vi "niDTS BT UTIL Parameters to Recepie.vi"(10 "BT Tx Parameters":T1={"Channel"=0, "Data Rate "=1, "Dut Tx Power"=0.0, "External Attenuation (dB)"=[0.0, 0.0, 0.0, 0.0], "Auto Level"=FALSE, "Packet type"=enum."DH1", "Payload Pattern"=enum."PN9", "Burst Sync"=enum."PREamble", "BD ADDRESS"=0, "Packet Length, bytes"=37, "ModAcc Measurement Paramaters"={"ModAcc Enable"=FALSE, "CFO Enable"=FALSE, "Character Select"=enum."DF1", "Averages"=1, "Averaging Mode"=enum."RMS", "Measurement Length"=-1, "Measurement Offset"=0}, "OBW Measurement Parameters"={"OBW Enable"=FALSE, "OBW Averages"=1, "Averaging Type"=enum."RMS", "Measurement Interval Mode"=enum."AUTO", "Measurement Interval Length (sec)"=0.005}, "TXP Measurement Parameters"={"TXP Power Enable"=FALSE, "TXP Averages"=1, "Averaging Type"=enum."RMS"}, "IBE  Measurement Parameters"={"IBE Enable"=FALSE, "IBE Averages"=1, "Averaging Type"=enum."RMS", "Numbe of Channels"=11, "Channel Mode"=enum."Centered", "Measurement Interval Mode"=enum."AUTO", "Measurement Interval Length (sec)"=0.005}, "Trace Enable"=FALSE, "Trigger"={"MinQuietTimeDuration (sec)"=0.0001, "TriggerDelay (sec)"=0.0, "TriggerEdge"=enum."RISing", "TriggerSource"=enum."RF0", "TriggerThreshold (dB)"=-20.0, "TriggerTimeout (sec)"=10.0}} {"BD ADDRESS" max=16777215 format="%.0x"}) -> (2 "BT Tx Parameters Out":T1={"Channel"=0, "Data Rate "=1, "Dut Tx Power"=0.0, "External Attenuation (dB)"=[0.0, 0.0, 0.0, 0.0], "Auto Level"=FALSE, "Packet type"=enum."DH1", "Payload Pattern"=enum."PN9", "Burst Sync"=enum."PREamble", "BD ADDRESS"=0, "Packet Length, bytes"=-1, "ModAcc Measurement Paramaters"={"ModAcc Enable"=FALSE, "CFO Enable"=FALSE, "Character Select"=enum."DF1", "Averages"=1, "Averaging Mode"=enum."RMS", "Measurement Length"=-1, "Measurement Offset"=0}, "OBW Measurement Parameters"={"OBW Enable"=FALSE, "OBW Averages"=1, "Averaging Type"=enum."RMS", "Measurement Interval Mode"=enum."AUTO", "Measurement Interval Length (sec)"=0.005}, "TXP Measurement Parameters"={"TXP Power Enable"=FALSE, "TXP Averages"=1, "Averaging Type"=enum."RMS"}, "IBE  Measurement Parameters"={"IBE Enable"=FALSE, "IBE Averages"=1, "Averaging Type"=enum."RMS", "Numbe of Channels"=11, "Channel Mode"=enum."Centered", "Measurement Interval Mode"=enum."AUTO", "Measurement Interval Length (sec)"=0.005}, "Trace Enable"=FALSE, "Trigger"={"MinQuietTimeDuration (sec)"=0.0001, "TriggerDelay (sec)"=0.0, "TriggerEdge"=enum."RISing", "TriggerSource"=enum."RF0", "TriggerThreshold (dB)"=-20.0, "TriggerTimeout (sec)"=10.0}} {"BD ADDRESS" max=16777215 format="%.0x"}, 4 "Payloads":T3[](array[typedef]), 5 "Measurements":enum16{"Other", "DF1", "DF2"}[](array[ring]))   [LabVIEW 2015, in "niDTS BT.lvlib"]
uses:
  niDTS BT.lvlib
  Tests/Tx Test/Includes/niDTS BT Tx Test INC Parameters.ctl
  Includes/niDTS BT INC Packet Type.ctl
  Tests/Tx Test/Includes/niDTS BT Tx Test INC BD Payload Data.ctl
  Tests/Tx Test/Includes/niDTS BT Tx Test INC Modulation Characteristics.ctl
  Includes/niDTS BT INC OBW Measurement Parameters.ctl
  Includes/niDTS BT INC TXP Measurement Parameters.ctl
  Tests/EDR Tx Test/Includes/niDTS BT INC EDR IBE Measurement Parameters.ctl
  Includes/niDTS BT DUT INC Trigger.ctl
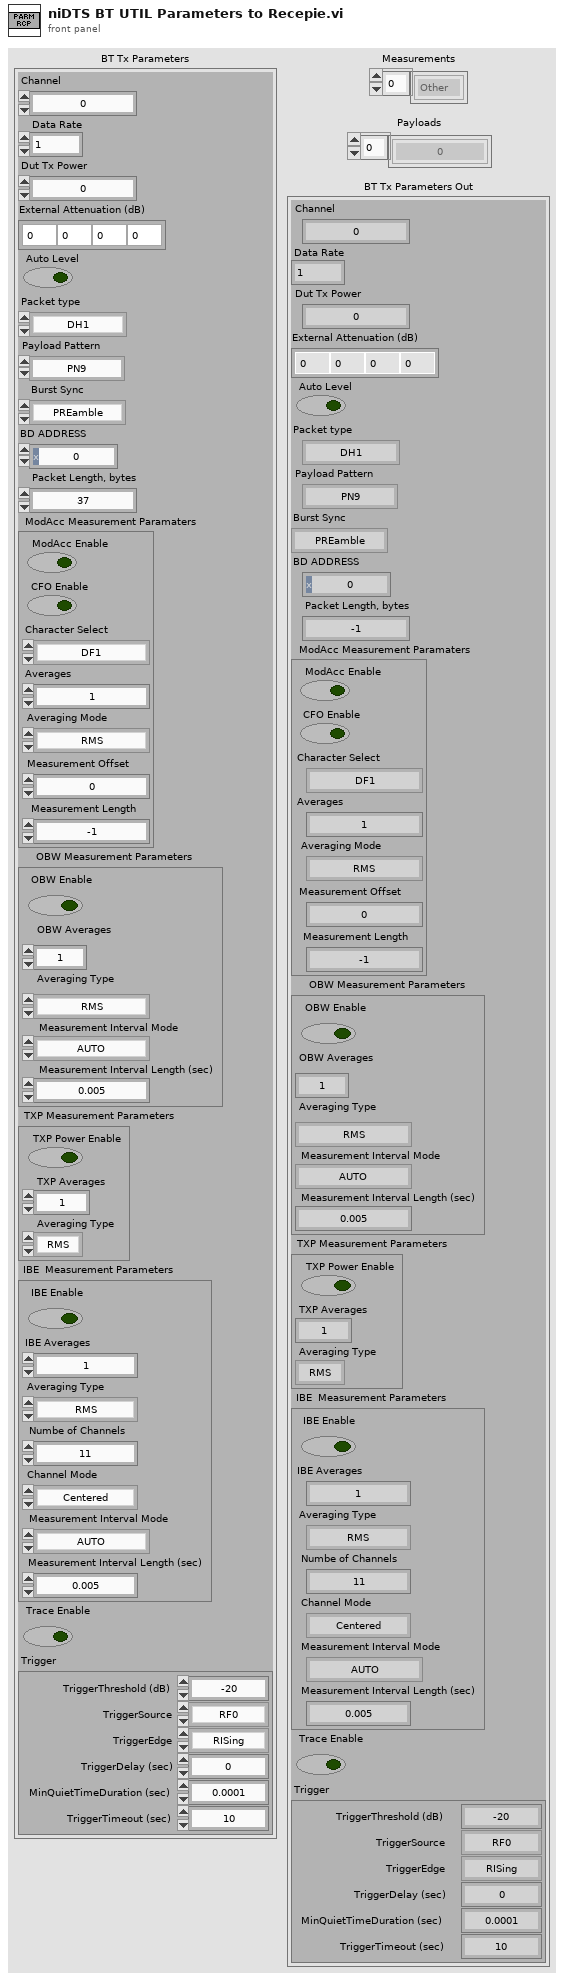
[diagram p1: front panel]
types:
  T1 = typedef "niDTS BT.lvlib/niDTS BT Tx Test INC Parameters.ctl" = cluster{"Channel":i32, "Data Rate ":i32, "Dut Tx Power":dbl, "External Attenuation (dB)":dbl[], "Auto Level":bool, "Packet type":T2, "Payload Pattern":T3, "Burst Sync":enum16{"NONE", "PREamble"}, "BD ADDRESS":u32, "Packet Length, bytes":i32, "ModAcc Measurement Paramaters":cluster{"ModAcc Enable":bool, "CFO Enable":bool, "Character Select":T4, "Averages":i32, "Averaging Mode":enum16{"RMS", "LOG", "SCALAR", "MAX", "MIN", "VECTOR"}, "Measurement Length":i32, "Measurement Offset":i32}, "OBW Measurement Parameters":T5, "TXP Measurement Parameters":T6, "IBE  Measurement Parameters":T7, "Trace Enable":bool, "Trigger":T8}
  T2 = typedef "niDTS BT.lvlib/niDTS BT INC Packet Type.ctl" = enum16{"NULL", "POLL", "FHS", "DM1", "DH1", "HV1", "HV2", "HV3", "EV3", "DV", "AUX1", "DM3", "DH3", "EV4", "EV5", "DM5", "DH5", "LE-TP"}
  T3 = typedef "niDTS BT.lvlib/niDTS BT Tx Test INC BD Payload Data.ctl" = enum16{"0", "1", "01", "00001111", "PN9", "AUTO"}
  T4 = typedef "niDTS BT.lvlib/niDTS BT Tx Test INC Modulation Characteristics.ctl" = enum16{"DF1", "DF2", "BOTH"}
  T5 = typedef "niDTS BT.lvlib/niDTS BT INC OBW Measurement Parameters.ctl" = cluster{"OBW Enable":bool, "OBW Averages":i32, "Averaging Type":enum16{"RMS", "LOG", "SCALAR", "MAX", "MIN", "VECTOR"}, "Measurement Interval Mode":enum16{"AUTO", "MANUAL"}, "Measurement Interval Length (sec)":dbl}
  T6 = typedef "niDTS BT.lvlib/niDTS BT INC TXP Measurement Parameters.ctl" = cluster{"TXP Power Enable":bool, "TXP Averages":i32, "Averaging Type":enum16{"RMS", "LOG", "SCALAR", "MAX", "MIN"}}
  T7 = typedef "niDTS BT.lvlib/niDTS BT INC EDR IBE Measurement Parameters.ctl" = cluster{"IBE Enable":bool, "IBE Averages":i32, "Averaging Type":enum16{"RMS", "LOG", "SCALAR", "MAX", "MIN", "VECTOR"}, "Numbe of Channels":i32, "Channel Mode":enum16{"InBand", "Centered"}, "Measurement Interval Mode":enum16{"AUTO", "MANUAL"}, "Measurement Interval Length (sec)":dbl}
  T8 = typedef "niDTS BT.lvlib/niDTS BT DUT INC Trigger.ctl" = cluster{"MinQuietTimeDuration (sec)":dbl, "TriggerDelay (sec)":dbl, "TriggerEdge":enum16{"RISing", "FALLing"}, "TriggerSource":enum16{"IMMediate", "RF0", "PFI0", "PFI1", "RTS0", "RTS1", "RTS2", "RTS3", "RTS4", "RTS5", "RTS6", "RTS7", "PXIStar", "SOFT"}, "TriggerThreshold (dB)":dbl, "TriggerTimeout (sec)":dbl}
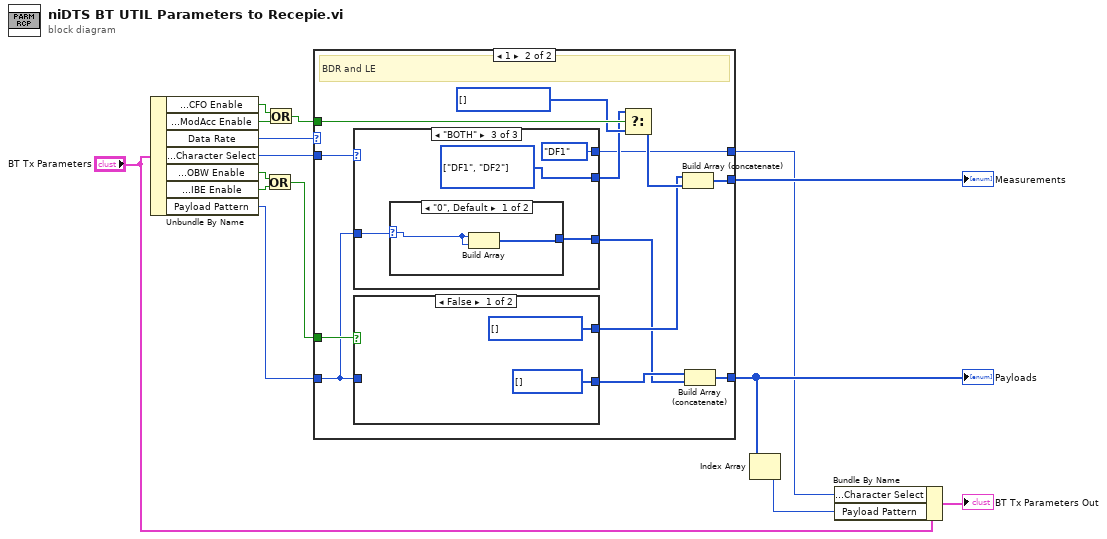
[diagram p0: block diagram]
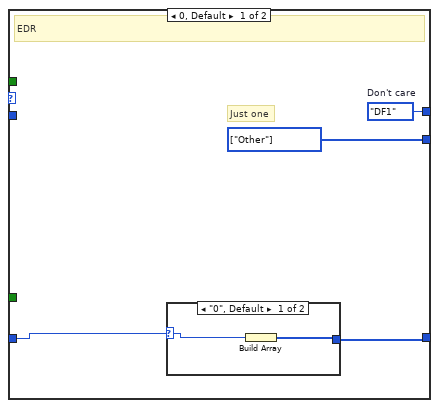
[diagram p2: hidden frame]
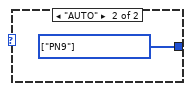
[diagram p3: hidden frame]
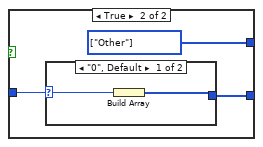
[diagram p4: hidden frame]
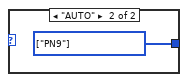
[diagram p5: hidden frame]
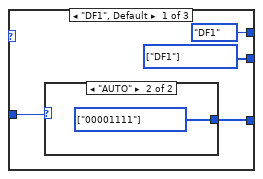
[diagram p6: hidden frame]
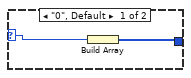
[diagram p7: hidden frame]
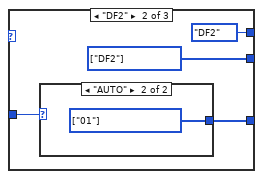
[diagram p8: hidden frame]
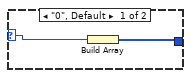
[diagram p9: hidden frame]
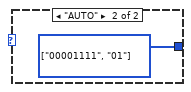
[diagram p10: hidden frame]
diagram:
  n1 = Unbundle By Name("BT Tx Parameters") -> ("ModAcc Measurement Paramaters.CFO Enable"=w2:bool, "ModAcc Measurement Paramaters.ModAcc Enable"=w3:bool, "Data Rate"=w15:i32, "ModAcc Measurement Paramaters.Character Select"=w14:T4, "OBW Measurement Parameters.OBW Enable"=w13:bool, "IBE  Measurement Parameters.IBE Enable"=w12:bool, "Payload Pattern"=w9:T3)
  n2 = Or(x=w13, y=w12) -> (x .or. y?=w11:bool)
  n3 = Or(x=w2, y=w3) -> (x .or. y?=w1:bool)
  n4 = case shown="1" w15 {
    tunnel: w14 -> [_ w35]
    tunnel: [w19 w34] -> w10
    tunnel: w11 -> [_ w29]
    tunnel: w1 -> [_ w33]
    tunnel: w9 -> [w17 w26]
    tunnel: [w18 w24] -> w8
    tunnel: [w16 w23] -> w4
    frame 0, Default {
      w16 = niDTS_BT_Tx_Test_INC_Modulation_Characteristics."DF1"  # Don't care
      w19 = enum16{"Other", "DF1", "DF2"}[] [enum."Other"] items=["Other", "DF1", "DF2"]
      # "Just one"
      # "EDR"
      n5 = case shown="\"0\", Default" w17 {
        selector: w17 -> [w21 _]
        tunnel: [w20 w22] -> w18
        frame "0", Default {
          n6 = Build Array(w21) -> (w20:T3[])
        }
        frame "AUTO" {
          w22 = T3[] [enum."PN9"] items=["0", "1", "01", "00001111", "PN9", "AUTO"]
        }
      }
    }
    frame 1 {
      w32 = enum16{"Other", "DF1", "DF2"}[] [] items=["Other", "DF1", "DF2"]
      # "BDR and LE"
      n7 = case shown="\"BOTH\"" w35 {
        tunnel: [w47 w54 w60] -> w31
        tunnel: w26 -> [w46 w53 w61]
        tunnel: [w45 w52 w59] -> w25
        tunnel: [niDTS_BT_Tx_Test_INC_Modulation_Characteristics."DF1" ("Character Select") niDTS_BT_Tx_Test_INC_Modulation_Characteristics."DF2" ("Character Select") niDTS_BT_Tx_Test_INC_Modulation_Characteristics."DF1" ("Character Select")] -> w23
        frame "DF1", Default {
          w47 = enum16{"Other", "DF1", "DF2"}[] [enum."DF1"] items=["Other", "DF1", "DF2"]
          n8 = case shown="\"AUTO\"" w46 {
            selector: w46 -> [w49 _]
            tunnel: [w48 w50] -> w45
            frame "0", Default {
              n9 = Build Array(w49) -> (w48:T3[])
            }
            frame "AUTO" {
              w50 = T3[] [enum."00001111"] items=["0", "1", "01", "00001111", "PN9", "AUTO"]
            }
          }
        }
        frame "DF2" {
          w54 = enum16{"Other", "DF1", "DF2"}[] [enum."DF2"] items=["Other", "DF1", "DF2"]
          n10 = case shown="\"AUTO\"" w53 {
            selector: w53 -> [w56 _]
            tunnel: [w55 w57] -> w52
            frame "0", Default {
              n11 = Build Array(w56) -> (w55:T3[])
            }
            frame "AUTO" {
              w57 = T3[] [enum."01"] items=["0", "1", "01", "00001111", "PN9", "AUTO"]
            }
          }
        }
        frame "BOTH" {
          w60 = enum16{"Other", "DF1", "DF2"}[] [enum."DF1", enum."DF2"] items=["Other", "DF1", "DF2"]
          n12 = case shown="\"0\", Default" w61 {
            selector: w61 -> [w62 _]
            tunnel: [w63 w64] -> w59
            frame "0", Default {
              n13 = Build Array(w62, w62) -> (w63:T3[])
            }
            frame "AUTO" {
              w64 = T3[] [enum."00001111", enum."01"] items=["0", "1", "01", "00001111", "PN9", "AUTO"]
            }
          }
        }
      }
      n14 = case shown="False" w29 {
        tunnel: [w36 w40] -> w28
        tunnel: [w37 w39] -> w27
        tunnel: w26 -> [_ w38]
        frame False {
          w36 = T3[] [] items=["0", "1", "01", "00001111", "PN9", "AUTO"]
          w37 = enum16{"Other", "DF1", "DF2"}[] [] items=["Other", "DF1", "DF2"]
        }
        frame True {
          w39 = enum16{"Other", "DF1", "DF2"}[] [enum."Other"] items=["Other", "DF1", "DF2"]
          n15 = case shown="\"0\", Default" w38 {
            selector: w38 -> [w42 _]
            tunnel: [w41 w43] -> w40
            frame "0", Default {
              n16 = Build Array(w42) -> (w41:T3[])
            }
            frame "AUTO" {
              w43 = T3[] [enum."PN9"] items=["0", "1", "01", "00001111", "PN9", "AUTO"]
            }
          }
        }
      }
      n17 = Select(t=w31, s=w33, f=w32) -> (s? t:f=w30:enum16{"Other", "DF1", "DF2"}[])
      n18 = Build Array (concatenate)(w27, w30) -> (w34:enum16{"Other", "DF1", "DF2"}[])
      n19 = Build Array (concatenate)(w28, w25) -> (w24:T3[])
    }
  }
  "Measurements" <- w10
  "Payloads" <- w8
  n20 = Index Array(array=w8) -> (element=w6:T3)  [unwired: 1 in]
  n21 = Bundle By Name(cluster="BT Tx Parameters", "ModAcc Measurement Paramaters.Character Select"=w4, "Payload Pattern"=w6) -> (→"BT Tx Parameters Out":T1)
